vi "ASI_wait_for_task_DONE.vi"(1 "error in":errorcluster) -> (0 "error out":errorcluster)   [LabVIEW 2015]
uses:
  <vilib>/Utility/error.llb/DialogType.ctl
  GLOBAL/Global_ASI_stage.vi
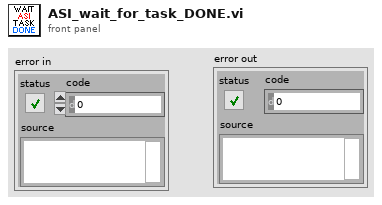
[diagram p1: front panel]
types:
  T1 = typedef "DialogType.ctl" = u16
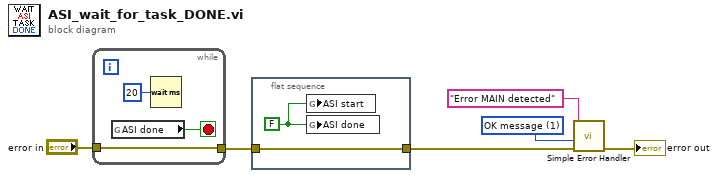
[diagram p0: block diagram]
diagram:
  w2 = T1 1 items=["no dialog", "OK message", "continue or stop message", "OK message + warnings", "continue/stop + warnings"] ("type of dialog (OK msg:1)")
  n1 = while {
    tunnel: "error in" -> [w8]
    tunnel: [w8] -> w5
    stop <- w9 stop-if-true
    n2 = global read "Global_ASI_stage.vi" "ASI done"() -> (w9:bool)
    n3 = Wait (ms)(milliseconds to wait=u32 20) -> ()  [unwired: 1 out]
  }
  n4 = flat-sequence {
    tunnel: [w10] -> w4
    tunnel: w5 -> [w10]
    frame #0 {
      w11 = FALSE ("ANDOR done")
      n5 = global write "Global_ASI_stage.vi" "ASI start"(w11) -> ()
      n6 = global write "Global_ASI_stage.vi" "ASI done"(w11) -> ()
    }
  }
  n7 = call <vilib>:"Simple Error Handler.vi"("error source (\" \")"="Error MAIN detected" ("error source (\" \")"), "type of dialog (OK msg:1)"=w2, "error in (no error)"=w4) -> ("error out"=→"error out":errorcluster)  [unwired: 2 in, 4 out]
